vi "FTW-Example-PubSubSockets.vi"() -> ()   [LabVIEW 2015]
uses:
  source/actor/Message/Base/FTW-Message.lvclass
  source/actor/Ether/FTW-Ether.lvclass
  source/actor/Publisher/FTW-Publisher.lvclass
  source/actor/Subscriber/FTW-Subscriber.lvclass
panel:
  out "Sender Identity 2":string
  out "Sender Identity":string
  out "Elapsed Time":dbl format="%.6fsec"
  in  "Connection":string(combo)="inproc://*"
  out "Request Body 2":string
  out "Request Header 2":string
  out "Request Body":string
  out "Request Header":string
  out "Timed out?":bool
  out "Actual Server Address":string
  out "error out":errorcluster
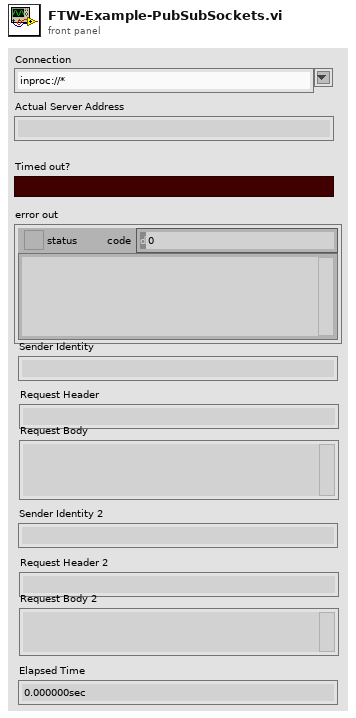
[diagram p1: front panel]
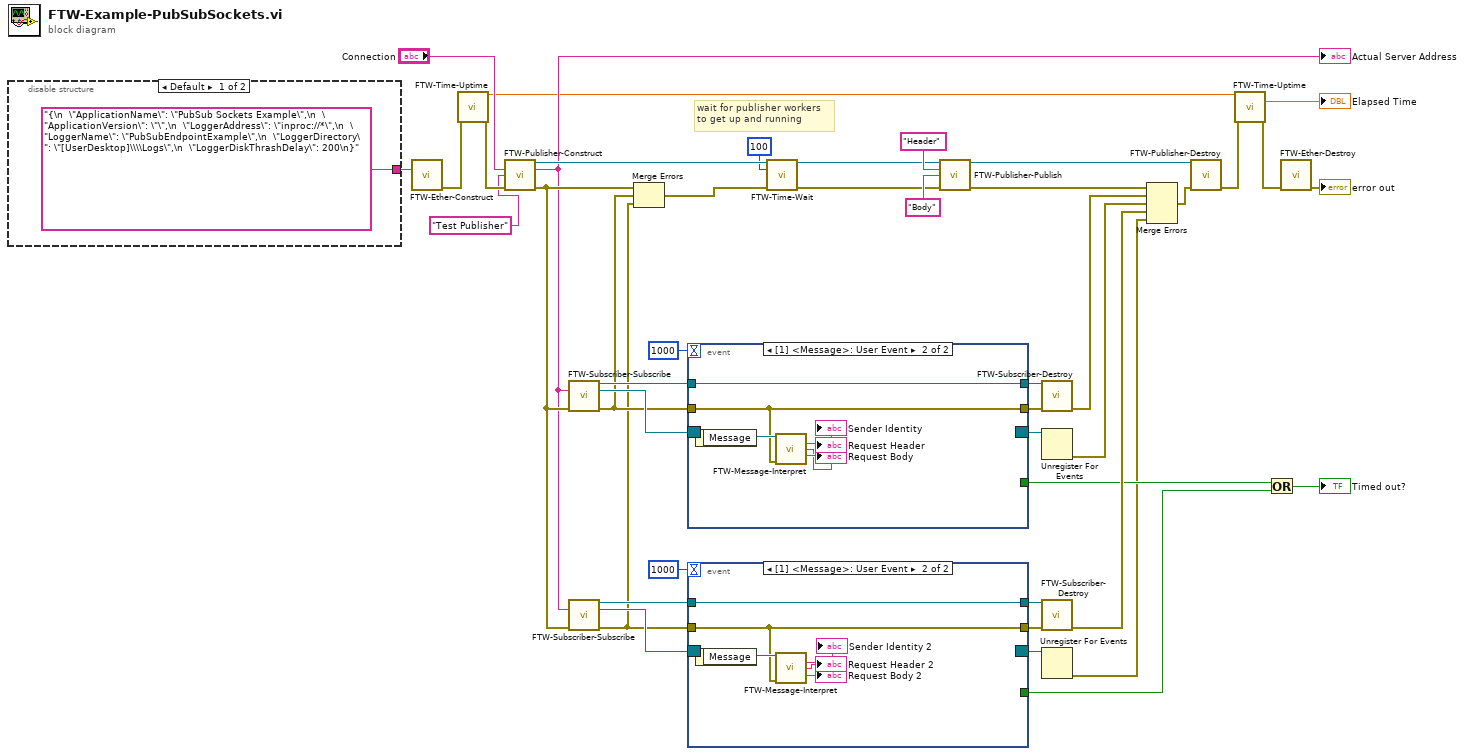
[diagram p0: block diagram]
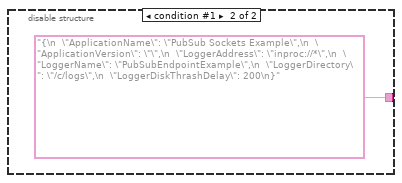
[diagram p2: hidden frame]
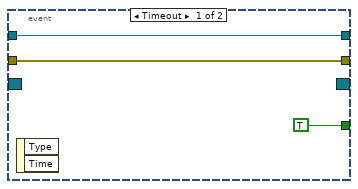
[diagram p3: hidden frame]
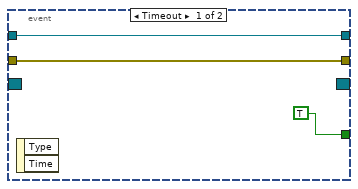
[diagram p4: hidden frame]
diagram:
  # "wait for publisher workers\nto get up and running"
  n1 = disable-structure shown="Default" {
    disable-tunnel: ["{\n  \"ApplicationName\": \"PubSub Sockets Example\",\n  \"ApplicationVersion\": \"\",\n  \"LoggerAddress\": \"inproc://*\",\n  \"LoggerName\": \"PubSubEndpointExample\",\n  \"LoggerDirectory\": \"[UserDesktop]\\\\Logs\",\n  \"LoggerDiskThrashDelay\": 200\n}" ("FTW Ether Configuration") "{\n  \"ApplicationName\": \"PubSub Sockets Example\",\n  \"ApplicationVersion\": \"\",\n  \"LoggerAddress\": \"inproc://*\",\n  \"LoggerName\": \"PubSubEndpointExample\",\n  \"LoggerDirectory\": \"/c/logs\",\n  \"LoggerDiskThrashDelay\": 200\n}" ("FTW Ether Configuration")] -> w39
    frame condition #0 (active) {
    }
    frame condition #1 {
    }
  }
  n2 = call "FTW-Ether-Construct.vi"("FTW Ether Configuration"=w39) -> ("error out"=w37:errorcluster)  [unwired: 14 in]
  n3 = call "FTW-Time-Uptime.vi"("error in"=w37) -> ("Current Uptime"=w3:dbl, "error out"=w4:errorcluster)  [unwired: 12 in, 1 out]
  n4 = call "FTW-Publisher-Construct.vi"("Address"="Connection", "Identity"="Test Publisher", "error in"=w4) -> ("FTW-Publisher Out"=w33:refnum<class "FTW-Publisher.lvclass">, "Actual Address"=w29:string, "error out"=w30:errorcluster)  [unwired: 10 in]
  "Actual Server Address" <- w29
  n5 = call "FTW-Subscriber-Subscribe.vi"("Addresses"=w29, "error in"=w30) -> ("FTW-Subscription Out"=w35:refnum<class "FTW-Subscriber.lvclass">, "Subscriber Registration"=w36:refnum<event-registration>, "error out"=w27:errorcluster)  [unwired: 11 in]
  n6 = call "FTW-Subscriber-Subscribe.vi"("Addresses"=w29, "error in"=w30) -> ("FTW-Subscription Out"=w32:refnum<class "FTW-Subscriber.lvclass">, "Subscriber Registration"=w31:refnum<event-registration>, "error out"=w26:errorcluster)  [unwired: 11 in]
  n7 = Merge Errors(w30, w27, w26) -> (w28:errorcluster)
  n8 = event shown="[1] <Message>: User Event" {
    selector: w36 -> [_ _]
    dyn-events: [_ _] -> w10
    timeout: 1000 -> [_ _]
    tunnel: w35 -> [w47 w52]
    tunnel: w27 -> [w46 w51]
    tunnel: [w47 w52] -> w25
    tunnel: [w46 w51] -> w24
    tunnel: [TRUE _] -> w13
    event Timeout {
      n9 = event-data() -> ()  [unwired: 1 in, 2 out]
    }
    event User Event {
      n10 = event-data() -> ("Message"=w53:refnum<class "FTW-Message.lvclass">)  [unwired: 1 in]
      n11 = call-dynamic "FTW-Message-Interpret.vi"("FTW Message"=w53, "error in"=w51) -> ("Sender Identity"=→"Sender Identity":string, "Message Header"=→"Request Header":string, "Message Body"=→"Request Body":string)  [unwired: 9 in, 2 out]
    }
  }
  n12 = event shown="[1] <Message>: User Event" {
    selector: w31 -> [_ _]
    dyn-events: [_ _] -> w9
    timeout: 1000 -> [_ _]
    tunnel: w32 -> [w56 w61]
    tunnel: w26 -> [w55 w60]
    tunnel: [w56 w61] -> w23
    tunnel: [w55 w60] -> w22
    tunnel: [TRUE _] -> w11
    event Timeout {
      n13 = event-data() -> ()  [unwired: 1 in, 2 out]
    }
    event User Event {
      n14 = event-data() -> ("Message"=w62:refnum<class "FTW-Message.lvclass">)  [unwired: 1 in]
      n15 = call-dynamic "FTW-Message-Interpret.vi"("FTW Message"=w62, "error in"=w60) -> ("Sender Identity"=→"Sender Identity 2":string, "Message Header"=→"Request Header 2":string, "Message Body"=→"Request Body 2":string)  [unwired: 9 in, 2 out]
    }
  }
  n16 = call "FTW-Time-Wait.vi"("Wait Time (ms)"=u32 100, "error in"=w28) -> ("error out"=w15:errorcluster)  [unwired: 13 in]
  n17 = call "FTW-Publisher-Publish.vi"("FTW-Publisher In"=w33, "Header"="Header" ("Message Header"), "Body"="Body" ("Message Body"), "error in"=w15) -> ("FTW-Publisher Out"=w18:refnum<class "FTW-Publisher.lvclass">, "error out"=w34:errorcluster)  [unwired: 10 in]
  n18 = call "FTW-Subscriber-Destroy.vi"("FTW-Subscription In"=w25, "error in"=w24) -> ("error out"=w21:errorcluster)  [unwired: 13 in]
  n19 = Unregister For Events(event registration refnum=w10) -> (error out=w8:errorcluster)  [unwired: 1 in]
  n20 = call "FTW-Subscriber-Destroy.vi"("FTW-Subscription In"=w23, "error in"=w22) -> ("error out"=w20:errorcluster)  [unwired: 13 in]
  n21 = Unregister For Events(event registration refnum=w9) -> (error out=w7:errorcluster)  [unwired: 1 in]
  n22 = Merge Errors(w34, w21, w8, w20, w7) -> (w40:errorcluster)
  n23 = call "FTW-Publisher-Destroy.vi"("FTW-Publisher In"=w18, "error in"=w40) -> ("error out"=w19:errorcluster)  [unwired: 13 in]
  n24 = call "FTW-Time-Uptime.vi"("Previous Uptime"=w3, "error in"=w19) -> ("Elapsed Time"=→"Elapsed Time":dbl, "error out"=w5:errorcluster)  [unwired: 11 in, 1 out]
  n25 = Or(x=w13, y=w11) -> (x .or. y?=→"Timed out?":bool)
  n26 = call "FTW-Ether-Destroy.vi"("error in"=w5) -> ("error out"=→"error out":errorcluster)  [unwired: 14 in]
